vi "Wait for Files.vi"(6 "Timeout (sec)":u32=60, 8 "Error In":errorcluster, 9 "# of Files in Directory":i32=2, 10 "Log Directory":path, 11 "TestCase in":refnum<class "TestCase.lvclass">) -> (0 "Error Out":errorcluster, 3 "TestCase out":refnum<class "TestCase.lvclass">)   [LabVIEW 2027, in "Embedded Data Logger Windows System Tests.lvclass"]
uses:
  Embedded Data Logger Windows System Tests.lvclass
  <vilib>/addons/_JKI Toolkits/VI Tester/TestCase.llb/TestCase.lvclass
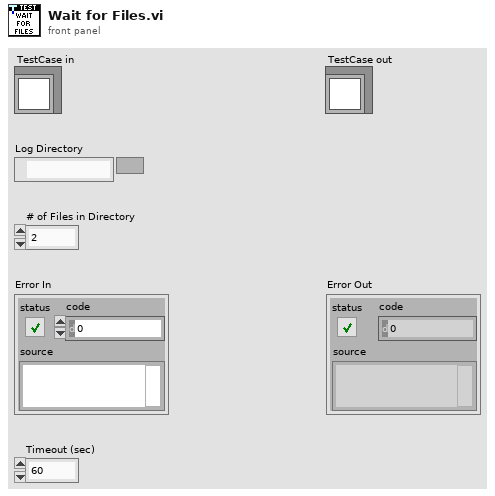
[diagram p1: front panel]
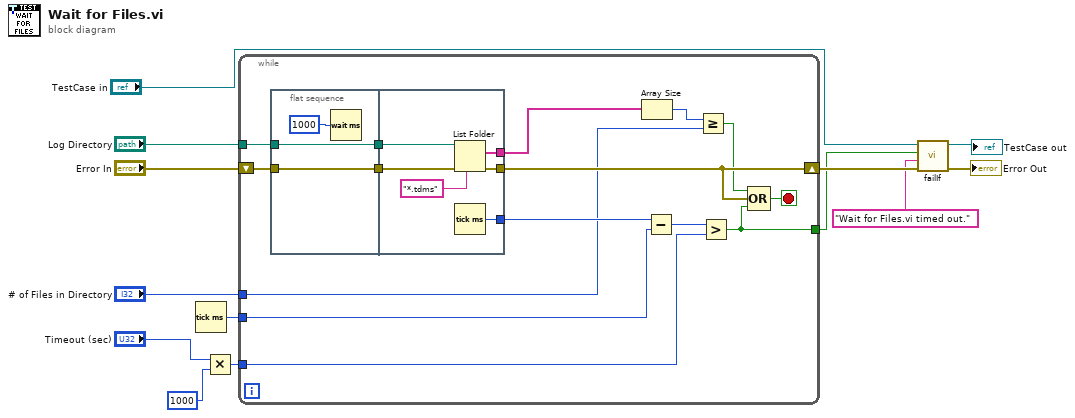
[diagram p0: block diagram]
diagram:
  n1 = Tick Count (ms)() -> (millisecond timer value=w13:u32)
  n2 = Multiply(x="Timeout (sec)", y=u32 1000) -> (x*y=w8:u32)
  n3 = while {
    tunnel: w13 -> [w21]
    tunnel: "Log Directory" -> [w28]
    shift-right: [w18] -> w6
    shift-left: "Error In" -> [w27]
    tunnel: w8 -> [w16]
    tunnel: "# of Files in Directory" -> [w15]
    tunnel: [w14] -> w4
    stop <- w19 stop-if-true
    n4 = flat-sequence {
      tunnel: w27 -> [w30]
      tunnel: w28 -> [w31]
      tunnel: [w31] -> w26
      tunnel: [w30] -> w25
      tunnel: [w35] -> w18
      tunnel: w26 -> [w37]
      tunnel: w25 -> [w36]
      tunnel: [w33] -> w24
      tunnel: [w32] -> w20
      frame #0 {
        n5 = Wait (ms)(milliseconds to wait=u32 1000) -> ()  [unwired: 1 out]
      }
      frame #1 {
        n6 = List Folder(path=w37, pattern="*.tdms", error in=w36) -> (filenames=w33:string[], error out=w35:errorcluster)  [unwired: 1 in, 2 out]
        n7 = Tick Count (ms)() -> (millisecond timer value=w32:u32)
      }
    }
    n8 = Array Size(array=w24) -> (size(s)=w23:i32)
    n9 = Subtract(x=w20, y=w21) -> (x-y=w22:u32)
    n10 = Greater Or Equal?(x=w23, y=w15) -> (x >= y?=w17:bool)
    n11 = Greater?(x=w22, y=w16) -> (0:w14:bool)
    n12 = Compound Arithmetic op=OR(w17, w18, w14) -> (w19:bool)
  }
  n13 = call-dynamic "failIf.vi"("error in (no error)"=w6, "message (\"\")"="Wait for Files.vi timed out." ("message (\"\")"), "fail"=w4, "TestCase in"="TestCase in") -> ("error out"=→"Error Out":errorcluster, "TestCase out"=→"TestCase out":refnum<class "TestCase.lvclass">)  [unwired: 6 in]
